vi "myRIO_BRig_RT__MTrig_count.vi"(0 "input_dataMTrig":u16[](array[numeric])) -> (14 "output_dataMTrig":u16[](array[numeric]))   [LabVIEW 2014]
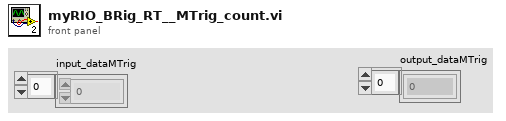
[diagram p1: front panel]
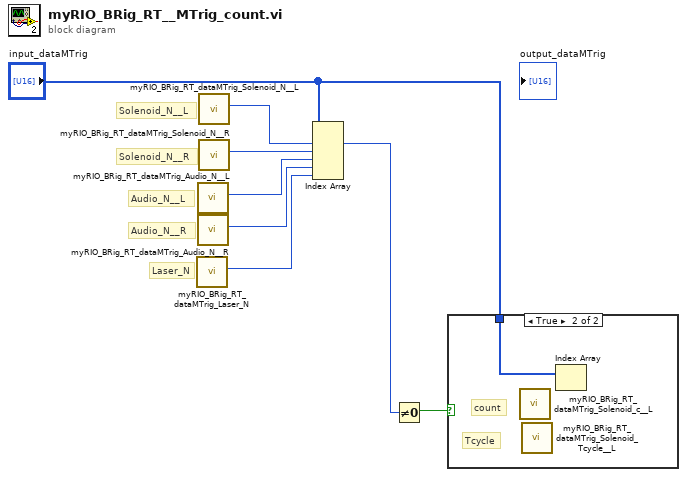
[diagram p0: block diagram]
diagram:
  # "Laser_N"
  # "Audio_N__R"
  # "Audio_N__L"
  # "Solenoid_N__R"
  # "Solenoid_N__L"
  n1 = call "myRIO_BRig_RT_dataMTrig_Laser_N.vi"() -> ("output_Laser_c"=w4:i32)  [unwired: 11 in]
  n2 = call "myRIO_BRig_RT_dataMTrig_Audio_N__L.vi"() -> ("output_Audio_N__L"=w6:i32)  [unwired: 11 in]
  n3 = call "myRIO_BRig_RT_dataMTrig_Audio_N__R.vi"() -> ("output_Audio_N__R"=w5:i32)  [unwired: 11 in]
  n4 = call "myRIO_BRig_RT_dataMTrig_Solenoid_N__L.vi"() -> ("output_Solenoid_N__L"=w8:i32)  [unwired: 11 in]
  n5 = call "myRIO_BRig_RT_dataMTrig_Solenoid_N__R.vi"() -> ("output_Solenoid_N__R"=w7:i32)  [unwired: 11 in]
  n6 = Index Array(array="input_dataMTrig", index #1=w8, index #2=w7, index #3=w6, index #4=w5, index #5=w4) -> (element #1=w3:u16)  [unwired: 4 out]
  n7 = Not Equal To 0?(x=w3) -> (x != 0?=w1:bool)
  n8 = case shown="True" w1 {
    tunnel: "input_dataMTrig" -> [_ w9]
    frame False {
    }
    frame True {
      # "Tcycle"
      # "count"
      n9 = call "myRIO_BRig_RT_dataMTrig_Solenoid_c__L.vi"() -> ()  [unwired: 11 in, 1 out]
      n10 = call "myRIO_BRig_RT_dataMTrig_Solenoid_Tcycle__L.vi"() -> ()  [unwired: 11 in, 1 out]
      n11 = Index Array(array=w9) -> ()  [unwired: 1 in, 1 out]
    }
  }
